vi "WPI_MotorControlClose.vi"(8 "error in":errorcluster, 11 "MotorControlDevRef":T1={"DeviceStatus"={"status"=FALSE, "code"=0, "source"=""}, "Type"=enum."PWM", "PWM"={"PWM Channel"=enum."Invalid", "DeadBand"={"Name"="", "maxPositivePwm"=0, "minPositivePwm"=0, "centerPwm"=0, "maxNegativePwm"=0, "minNegativePwm"=0, "angularRange"=0}}, "CAN"={"Device Number"=0, "SetOutput VI Ref"=variant(refnum<vi> refnum), "GetOutput VI Ref"=variant(refnum<vi> refnum), "Enable VI Ref"=variant(refnum<vi> refnum), "Disable VI Ref"=variant(refnum<vi> refnum), "Data"=variant}, "Invert"=FALSE, "DIO PWM"={"PWM \"Enable\" Channel"=enum."Invalid", "DIOChannel"=enum."Invalid", "PWM Rate"=0.0}}) -> (0 "error out":errorcluster)   [LabVIEW 2025]
doc: "Closes the reference to the motor controller you specify. Use this VI to close each motor control reference that you open with the Open VI.\n\nThis software is licensed. Open the labview\\readme\\WPI Robotics Library Open Source License.txt file for more information."
uses:
  <vilib>/Rock Robotics/WPI/MotorControl/WPI_MotorControlDeviceRef.ctl
  <vilib>/Rock Robotics/WPI/MotorControl/WPI_MotorControlType.ctl
  <vilib>/Rock Robotics/SystemInterfaces/DIO/FPGA_DIOPWMChannel.ctl
  <vilib>/Rock Robotics/WPI/PWM/WPI_PWMDeadband.ctl
  <vilib>/Rock Robotics/SystemInterfaces/DIO/FPGA_DIOChannel.ctl
  <vilib>/Rock Robotics/WPI/PWM/WPI_PWMChannelCacheOp.ctl
  <instrlib>/DC Motor Controller/HAIOL/DC Motor Controller.lvclass
  <vilib>/Rock Robotics/WPI/DigitalOutput/WPI_DigitalOutputDevRef.ctl
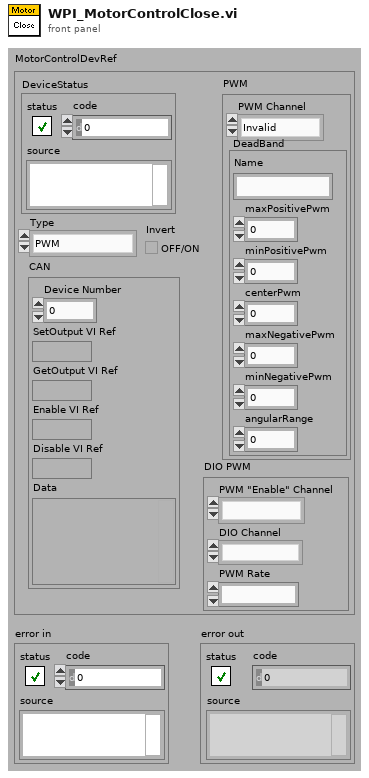
[diagram p1: front panel]
types:
  T1 = typedef "WPI_MotorControlDeviceRef.ctl" = cluster{"DeviceStatus":errorcluster, "Type":T2, "PWM":cluster{"PWM Channel":T3, "DeadBand":T4}, "CAN":cluster{"Device Number":u8, "SetOutput VI Ref":variant, "GetOutput VI Ref":variant, "Enable VI Ref":variant, "Disable VI Ref":variant, "Data":variant}, "Invert":bool, "DIO PWM":cluster{"PWM \"Enable\" Channel":T3, "DIOChannel":T5, "PWM Rate":dbl}}
  T2 = typedef "WPI_MotorControlType.ctl" = enum16{"PWM", "CAN", "DIO PWM"}
  T3 = typedef "FPGA_DIOPWMChannel.ctl" = enum8{"PWM 0", "PWM 1", "PWM 2", "PWM 3", "PWM 4", "PWM 5", "PWM 6", "PWM 7", "PWM 8", "PWM 9", "PWM MXP 0", "PWM MXP 1", "PWM MXP 2", "PWM MXP 3", "PWM MXP 4", "PWM MXP 5", "PWM MXP 6", "PWM MXP 7", "PWM MXP 8", "PWM MXP 9", "Invalid"}
  T4 = typedef "WPI_PWMDeadband.ctl" = cluster{"Name":string, "maxPositivePwm":i32, "minPositivePwm":i32, "centerPwm":i32, "maxNegativePwm":i32, "minNegativePwm":i32, "angularRange":u16}
  T5 = typedef "FPGA_DIOChannel.ctl" = enum8{"DIO 0", "DIO 1", "DIO 2", "DIO 3", "DIO 4", "DIO 5", "DIO 6", "DIO 7", "DIO 8", "DIO 9", "DIO MXP 0", "DIO MXP 1", "DIO MXP 2", "DIO MXP 3", "DIO MXP 4", "DIO MXP 5", "DIO MXP 6", "DIO MXP 7", "DIO MXP 8", "DIO MXP 9", "DIO MXP 10", "DIO MXP 11", "DIO MXP 12", "DIO MXP 13", "DIO MXP 14", "DIO MXP 15", "SPI Port CS1", "SPI Port CS2", "SPI Port CS3", "SPI Port MISO", "SPI Port MOSI", "Invalid"}
  T6 = typedef "WPI_DigitalOutputDevRef.ctl" = cluster{"DIO Channel":T5, "DevStatus":errorcluster}
  T7 = typedef "WPI_PWMChannelCacheOp.ctl" = enum16{"Acquire", "Release", "Status"}
  T8 = typedef "WPI_PWMDeviceRef.ctl" = cluster{"DeviceStatus":errorcluster, "PWM Channel":T3}
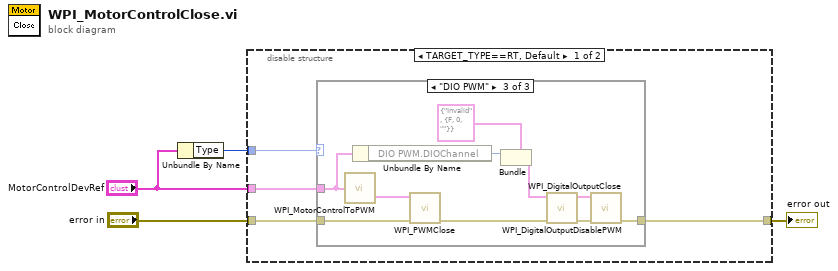
[diagram p0: block diagram]
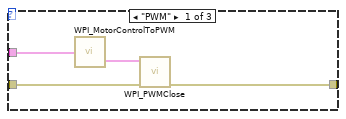
[diagram p2: hidden frame]
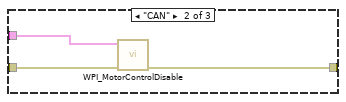
[diagram p3: hidden frame]
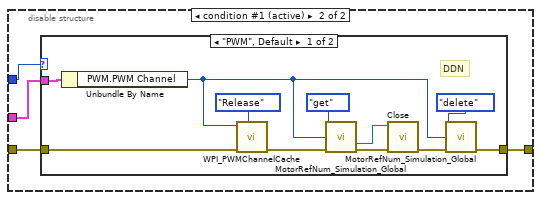
[diagram p4: hidden frame]
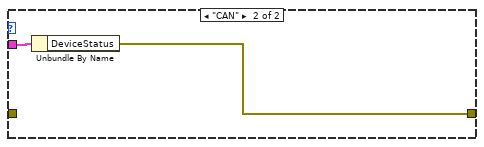
[diagram p5: hidden frame]
diagram:
  n1 = Unbundle By Name("MotorControlDevRef") -> ("Type"=w1:T2)
  n2 = disable-structure shown="TARGET_TYPE==RT, Default" {
    disable-tunnel: "error in" -> [w8 w28]
    disable-tunnel: [w7 w29] -> w3
    disable-tunnel: "MotorControlDevRef" -> [w6 w27]
    disable-tunnel: w1 -> [w5 w26]
    frame condition #0 {
      n3 = case shown="\"DIO PWM\"" w5 {
        tunnel: w8 -> [w12 w15 w25]
        tunnel: [w11 w14 w21] -> w7
        tunnel: w6 -> [w9 w13 w23]
        frame "PWM" {
          n4 = call <vilib>:"WPI_MotorControlToPWM.vi"("MotorControlDeviceRef"=w9) -> ("PWMDeviceRef"=w10:T8)  [unwired: 1 out]
          n5 = call <vilib>:"WPI_PWMClose.vi"("error in (no error)"=w12, "PWMDeviceRef"=w10) -> ("error out"=w11:errorcluster)  [unwired: 9 out]
        }
        frame "CAN" {
          n6 = call <vilib>:"WPI_MotorControlDisable.vi"("error in (no error)"=w15, "MotorControlDevRef"=w13) -> ("error out"=w14:errorcluster)  [unwired: 8 in, 1 out]
        }
        frame "DIO PWM" {
          n7 = call <vilib>:"WPI_MotorControlToPWM.vi"("MotorControlDeviceRef"=w23) -> ("PWMDeviceRef"=w24:T8)  [unwired: 1 out]
          n8 = Unbundle By Name(w23) -> ("DIO PWM.DIOChannel"=w20:T5)
          n9 = call <vilib>:"WPI_PWMClose.vi"("error in (no error)"=w25, "PWMDeviceRef"=w24) -> ("error out"=w16:errorcluster)  [unwired: 9 out]
          n10 = Bundle(cluster=T6 {"DIO Channel"=enum."Invalid", "DevStatus"={"status"=FALSE, "code"=0, "source"=""}} ("DigitalOutputDevRef"), "DIO Channel"=w20) -> (w17:T6)  [unwired: 1 in]
          n11 = call <vilib>:"WPI_DigitalOutputDisablePWM.vi"("error in (no error)"=w16, "DigitalOutputDevRef"=w17) -> ("error out"=w19:errorcluster, "DigitalOutputDevRef"=w18:T6)  [unwired: 8 in]
          n12 = call <vilib>:"WPI_DigitalOutputClose.vi"("error in (no error)"=w19, "DigitalOutputDevRef"=w18) -> ("error out"=w21:errorcluster)  [unwired: 9 in]
        }
      }
    }
    frame condition #1 (active) {
      n13 = case shown="\"PWM\", Default" w26 {
        tunnel: w28 -> [w32 _]
        tunnel: [w31 w41] -> w29
        tunnel: w27 -> [w40 w42]
        frame "PWM", Default {
          # "DDN"
          n14 = Unbundle By Name(w40) -> ("PWM.PWM Channel"=w33:T3)
          n15 = call <vilib>:"WPI_PWMChannelCache.vi"("Operation"=WPI_PWMChannelCacheOp."Release", "error in (no error)"=w32, "PWMChannel"=w33) -> ("error out"=w37:errorcluster)  [unwired: 2 in, 6 out]
          n16 = call <vilib>:"MotorRefNum_Simulation_Global.vi"("menu"=enum16{"set", "get", "delete"}."get", "PWM Channel"=w33, "error in (no error)"=w37) -> ("DC Motor Controller Get"=w30:refnum<class "DC Motor Controller.lvclass">, "error out"=w36:errorcluster)  [unwired: 11 in]
          n17 = call-dynamic "Close.vi"("error in (no error)"=w36, "DC Motor Controller in"=w30) -> ("error out"=w34:errorcluster)  [unwired: 9 in]
          n18 = call <vilib>:"MotorRefNum_Simulation_Global.vi"("menu"=enum16{"set", "get", "delete"}."delete", "PWM Channel"=w33, "error in (no error)"=w34) -> ("error out"=w31:errorcluster)  [unwired: 11 in, 1 out]
        }
        frame "CAN" {
          n19 = Unbundle By Name(w42) -> ("DeviceStatus"=w41:errorcluster)
        }
      }
    }
  }
  "error out" <- w3
